vi "graph_color_change.vi"() -> ()   [LabVIEW 2020]
uses:
  <vilib>/measure/NI_MABase.lvlib
panel:
  out "result":bool
  out "?":dynamicdata(graph)
  in  "stop":bool
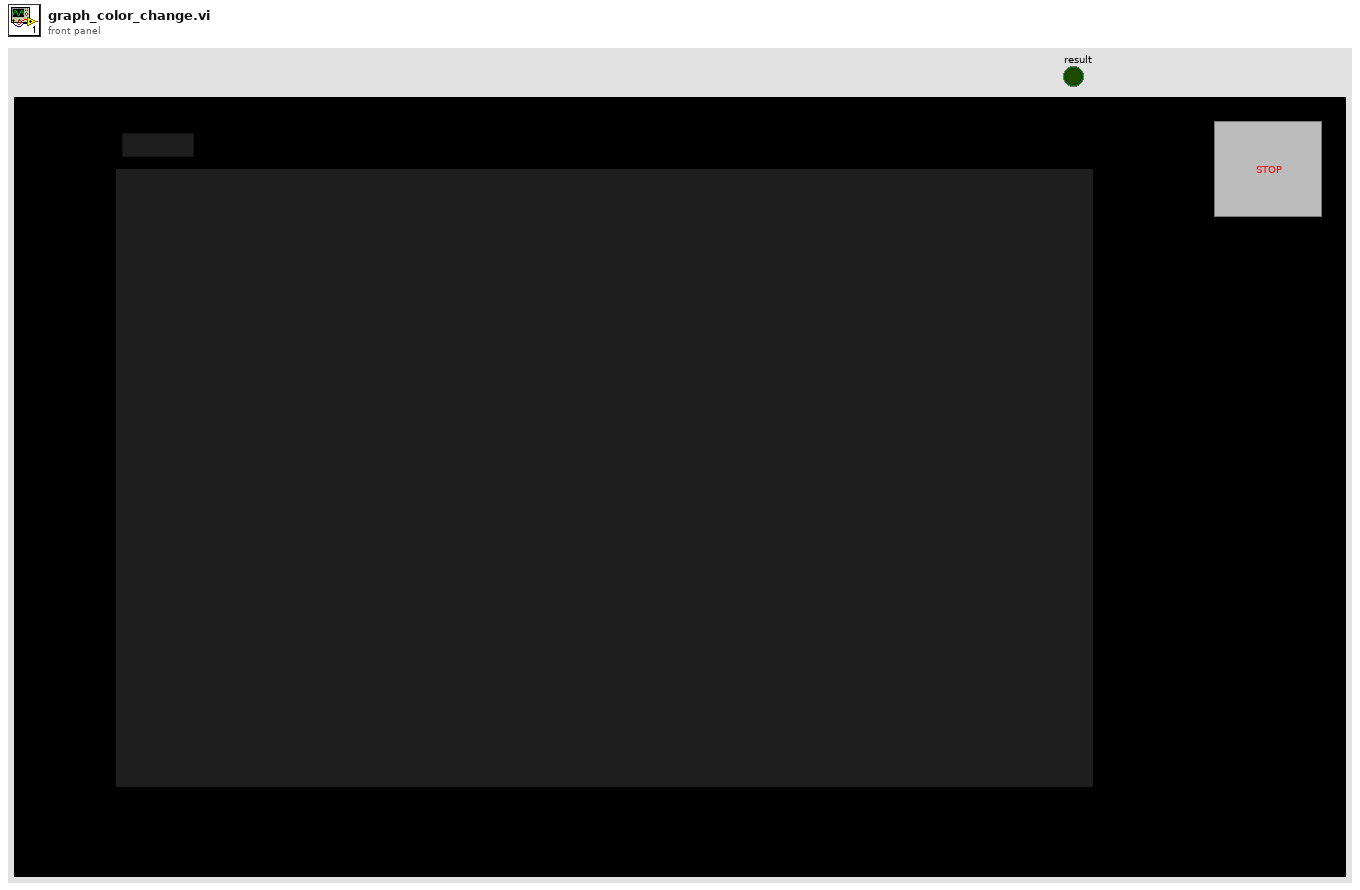
[diagram p1: front panel]
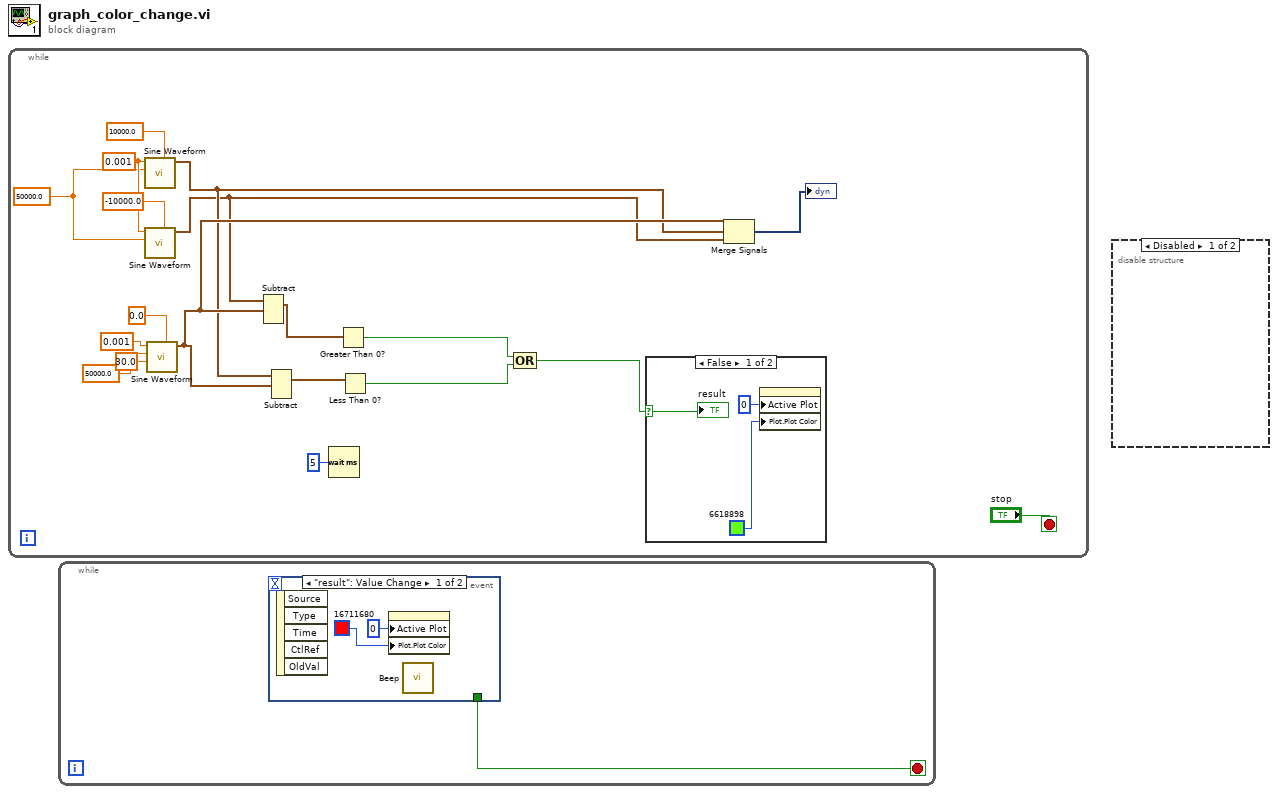
[diagram p0: block diagram]
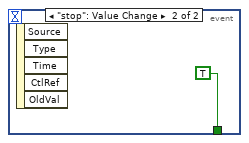
[diagram p3: hidden frame]
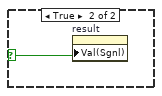
[diagram p4: hidden frame]
diagram:
  n1 = while {
    stop <- "stop" stop-if-true
    w10 = 50000.0 ("amplitude")
    w11 = 0.001 ("frequency")
    n2 = call <vilib>:"Sine Waveform.vi"("offset"=10000.0, "amplitude"=w10, "frequency"=w11) -> ("signal out"=w6:waveform(dbl))  [unwired: 7 in, 1 out]
    n3 = call <vilib>:"Sine Waveform.vi"("offset"=-10000.0, "amplitude"=w10, "frequency"=w11) -> ("signal out"=w5:waveform(dbl))  [unwired: 7 in, 1 out]
    n4 = call <vilib>:"Sine Waveform.vi"("offset"=0.0, "phase"=30.0, "amplitude"=50000.0, "frequency"=0.001) -> ("signal out"=w7:waveform(dbl))  [unwired: 6 in, 1 out]
    n5 = Subtract(1:w7, 2:w5) -> (0:w15:waveform(dbl))  [unwired: 1 in, 1 out]
    n6 = Subtract(1:w7, 2:w6) -> (0:w13:waveform(dbl))  [unwired: 1 in, 1 out]
    n7 = Wait (ms)(milliseconds to wait=u32 5) -> ()  [unwired: 1 out]
    n8 = Greater Than 0?(x=w15) -> (x > 0?=w14:bool)
    n9 = Less Than 0?(x=w13) -> (x < 0?=w12:bool)
    n10 = Compound Arithmetic op=OR(w14, w12) -> (w1:bool)
    n11 = case shown="False" w1 {
      selector: w1 -> [w22 w23]
      frame False {
        n12 = property class="WFChart (strict)"("Active Plot"=u32 0, "Plot.Plot Color"=u32 6618898) -> ()  [unwired: 2 in, 2 out]
        "result" <- w22
      }
      frame True {
        n13 = property on="result" class="Bool (strict)"("Val(Sgnl)"=w23) -> ()  [unwired: 2 in, 2 out]
      }
    }
    n14 = Merge Signals(w7, w6, w5) -> (→"?":dynamicdata)
  }
  n15 = while {
    stop <- w24 stop-if-true
    n16 = event shown="[0] \"result\": Value Change" {
      selector: _ -> [_ _]
      dyn-events: _ -> [_ _]
      timeout: _ -> [_ _]
      tunnel: [_ TRUE] -> w24
      event "result": Value Change {
        n17 = event-data() -> ()  [unwired: 1 in, 5 out]
        n18 = property class="WFChart (strict)"("Active Plot"=u32 0, "Plot.Plot Color"=u32 16711680) -> ()  [unwired: 2 in, 2 out]
        n19 = call <vilib>:"Beep.vi"() -> ()  [unwired: 12 in]
      }
      event "stop": Value Change {
        n20 = event-data() -> ()  [unwired: 1 in, 5 out]
      }
    }
  }
  n21 = disable-structure shown="Disabled" {
    frame Disabled {
    }
    frame Enabled {
    }
  }
